vi "Get Active Neurons.vi"(11 "Grid in":refnum<class "Grid.lvclass">) -> (2 "Position Neuron Active":u32[](array[numeric]), 3 "Grid out":refnum<class "Grid.lvclass">)   [LabVIEW 2016, in "Grid.lvclass"]
doc: "This method gets the IDs of all the nodes(neurons) that are active in the Grid"
uses:
  Grid.lvclass
  Grid.lvclass/Grid.ctl
  Neuron/Neuron.lvclass/Neuron.ctl
  Neuron/Neuron.lvclass
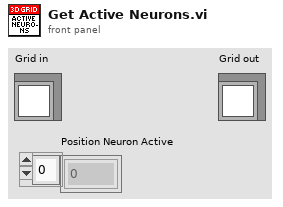
[diagram p1: front panel]
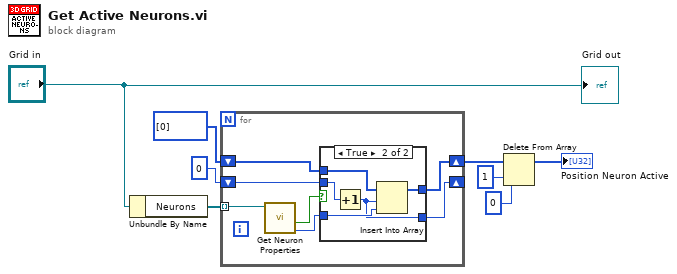
[diagram p0: block diagram]
diagram:
  n1 = Unbundle By Name("Grid in") -> ("Neurons"=w7:refnum<class "Neuron.lvclass">[])
  n2 = for {
    tunnel: w7 -> [w15] mode=indexing
    shift-right: [w13] -> w4
    shift-left: u32[] [0] -> [w12]
    shift-right: [w10] -> _
    shift-left: u32 0 ("ID") -> [w11]
    n3 = call "Get Neuron Properties.vi"("Neuron in"=w15) -> ("Position Key"=w14:i32, "Active"=w9:bool)  [unwired: 5 in, 4 out]
    n4 = case shown="True" w9 {
      tunnel: w14 -> [_ w22]
      tunnel: [w17 w21] -> w13
      tunnel: w12 -> [w17 w20]
      tunnel: w11 -> [w16 w19]
      tunnel: [w16 w18] -> w10
      frame False {
      }
      frame True {
        n5 = Increment(x=w19) -> (x+1=w18:u32)
        n6 = Insert Into Array(array=w20, index=w18, new element=w22) -> (w21:u32[])
      }
    }
  }
  n7 = Delete From Array(array=w4, length=1, index=0) -> (array with subset deleted=→"Position Neuron Active":u32[])  [unwired: 1 out]
  "Grid out" <- "Grid in"
